vi "binPixels.vi"(0 "pixel binning":u16(ring)=1 items=["1x1"=1, "2x2"=2, "4x4"=4, "8x8"=8, "16x16"=16], 1 "sCMOS cluster":cluster{"init":i16, "sCMOS handle":u32}) -> ()   [LabVIEW 2015]
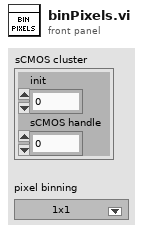
[diagram p1: front panel]
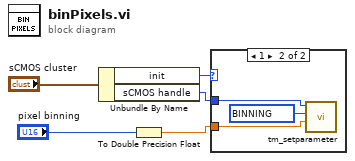
[diagram p0: block diagram]
diagram:
  n1 = Unbundle By Name("sCMOS cluster") -> ("init"=w4:i16, "sCMOS handle"=w3:u32)
  n2 = To Double Precision Float(number="pixel binning") -> (double precision float=w1:dbl)
  n3 = case shown="1" w4 {
    tunnel: w3 -> [_ w8]
    tunnel: w1 -> [_ w6]
    frame 0, Default {
    }
    frame 1 {
      w7 = u32 4215968 items=["BINNING"=4215968, "BITS PER CHANNEL"=2, "ACTIVE VIEW INDEX"=3, "CCD MODE"=4, "SENSOR MODE"=5, "READOUT MODE"=6, "EXPOSURE TIME"=7, "CONTRAST GAIN"=8, "CONTRAST OFFSET"=9, "LIGHT MODE"=10, "SENSITIVITY"=11, "WHITE BALANCE"=12, "PHOTON IMAGING MODE"=13, "HIGH DYNAMIC RANGE MODE"=14, "TRIGGER SOURCE"=15, "TRIGGER ACTIVE"=16, "TRIGGER MODE"=17, "TRIGGER POLARITY"=18, "TRIGGER GLOBAL EXPOSURE"=19, "FIRST TRIGGER BEHAVIOR"=20, "TRIGGER TIMES"=21, "OUTPUT TRIGGER POLARITY"=22, "OUTPUT TRIGGER DELAY"=23, "OUTPUT TRIGGER PERIOD"=24, "TEMPERATURE"=25, "TEMPERATURE TARGET"=26, "SENSOR COOLER FAN"=27, "MECHANICAL SHUTTER"=28, "BACK FOCUS POSITION"=29, "FRAMEBUNDLE MODE"=30, "FRAMEBUNDLE NUMBER"=31, "LINEBUNDLE HEIGHT"=32, "TRIGGER CONNECTOR"=33, "IMAGE PIXEL TYPE"=34, "OUTPUT TRIGGER KIND"=35, "READOUT DIRECTION"=36, "CHANNEL SYNC"=37] ("Parameter")
      n4 = call <userlib>:"tm_setparameter.vi"("Value in"=w6, "Parameter"=w7, "Handle in"=w8) -> ()  [unwired: 7 in, 2 out]
    }
  }
